vi "ProdaNG.ProcessStepResult.New.vi"(8 "error in (no error)":errorcluster, 10 "ProcessStepResult":T1, 11 "dbHandle":i32) -> (0 "error out":errorcluster, 2 "ProcessStepResult out":T1, 3 "dbHandle":i32)   [LabVIEW 2016]
doc: "This function creates a new record from a prefilled ProcessStepResult structure. Additionally the mdTime in the according product is set the current time and the mdProcessStepId is set to the created id.\nParameter:\nhandle is an Integer, which is returned by the function Login() at the creation of a new connection.\nprocessStepResult is a pointer on a ProcessStepResult structure, which elements must be prefilled. The structure must be defined and filled in the calling program. Nearly all elements of the structure must be set to reasonable values. The element id is filled by the DLL with a new Id for the created record, if the returncode is 0. The element startTime is filled automatically with the current time by the DLL and the endTime is deleted. \nThe element statusId is of particular importance:\nIf this element is passed with the value -1, the DLL automatically sets the standard status 2 (in Process), while otherwise the returned status is set.\n\nReturncodes:\n0 No error \n< 0 ORACLE Error code\n 6 (ERROR_INVALID_HANDLE) in case of an invalid handle"
uses:
  Controls/ProdaNG.ProcessStepResult.ctl
  Controls/ProdaNG.ProcessStepResultSize.ctl
  prodllNG.dll
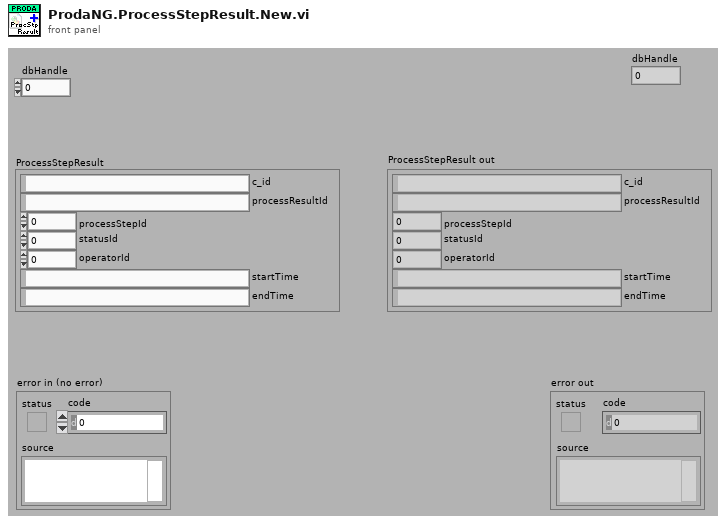
[diagram p1: front panel]
types:
  T1 = typedef "ProdaNG.ProcessStepResult.ctl" = cluster{"c_id":string, "processResultId":string, "processStepId":i32, "statusId":i32, "operatorId":i32, "startTime":string, "endTime":string}
  T2 = typedef "ProdaNG.ProcessStepResultSize.ctl" = cluster{"c_id":i32, "processResultId":i32, "processStepId":i32, "statusId":i32, "operatorId":i32, "startTime":i32, "endTime":i32}
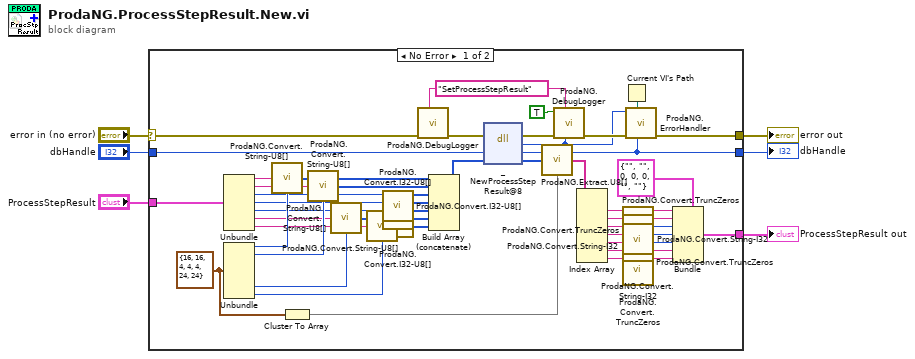
[diagram p0: block diagram]
diagram:
  n1 = case shown="No Error" "error in (no error)" {
    selector: "error in (no error)" -> [w31 w59]
    tunnel: [w28 w59] -> w5
    tunnel: "ProcessStepResult" -> [w29 _]
    tunnel: [w7 _] -> w3
    tunnel: "dbHandle" -> [w30 w58]
    tunnel: [w27 w58] -> w1
    frame No Error {
      w17 = T2 {"c_id"=16, "processResultId"=16, "processStepId"=4, "statusId"=4, "operatorId"=4, "startTime"=24, "endTime"=24} ("ProcessStepResultSize")
      w54 = "SetProcessStepResult" ("cmd")
      n2 = Unbundle(w29) -> ("c_id"=w56:string, "processResultId"=w57:string, "processStepId"=w44:i32, "statusId"=w43:i32, "operatorId"=w34:i32, "startTime"=w39:string, "endTime"=w38:string)
      n3 = Unbundle(w17) -> ("c_id"=w48:i32, "processResultId"=w46:i32, "startTime"=w33:i32, "endTime"=w32:i32)  [unwired: 3 out]
      n4 = call "ProdaNG.Convert.String-U8[].vi"("Input String"=w56, "Size"=w48) -> ("Output"=w47:u8[])
      n5 = Cluster To Array(cluster=w17) -> (array=w18:i32[])
      n6 = call "ProdaNG.Convert.String-U8[].vi"("Input String"=w57, "Size"=w46) -> ("Output"=w45:u8[])
      n7 = call "ProdaNG.Convert.String-U8[].vi"("Input String"=w39, "Size"=w33) -> ("Output"=w36:u8[])
      n8 = call "ProdaNG.Convert.String-U8[].vi"("Input String"=w38, "Size"=w32) -> ("Output"=w37:u8[])
      n9 = call "ProdaNG.Convert.I32-U8[].vi"("32bit integer"=w44) -> ("unsigned byte array"=w42:u8[])  [unwired: 10 in]
      n10 = call "ProdaNG.Convert.I32-U8[].vi"("32bit integer"=w43) -> ("unsigned byte array"=w41:u8[])  [unwired: 10 in]
      n11 = call "ProdaNG.Convert.I32-U8[].vi"("32bit integer"=w34) -> ("unsigned byte array"=w35:u8[])  [unwired: 10 in]
      n12 = call "ProdaNG.DebugLogger.vi"("cmd"=w54, "error in (no error)"=w31) -> ("error out"=w49:errorcluster)  [unwired: 9 in]
      n13 = Build Array (concatenate)(w47, w45, w42, w41, w35, w36, w37) -> (w40:u8[])
      n14 = dll-call lib="D:/svn/LineTraceSystem/SOFTWARE/sources/Database/ProdaNG/prodllNG.dll" fn="_NewProcessStepResult@8" ("ProDll.dll:InitProDll")(error in=w49, "dbHandle"=w30, "processResult"=w40) -> (error out=w52:errorcluster, "return type"=w50:i32, "dbHandle"=w27:i32, "processResult"=w19:u8[])  [unwired: 2 in, 1 out]
      n15 = call "ProdaNG.Extract.U8[].vi"("unsigned byte array"=w19, "Sizes"=w18) -> ("Elements"=w16:string[])
      n16 = call "ProdaNG.DebugLogger.vi"("return type"=w50, "cmd"=w54, "error in (no error)"=w52, "done? (F)"=TRUE) -> ("error out"=w51:errorcluster)  [unwired: 7 in]
      n17 = Index Array(array=w16) -> (element #1=w21:string, element #2=w20:string, element #3=w26:string, element #4=w10:string, element #5=w9:string, element #6=w11:string, element #7=w14:string)  [unwired: 7 in]
      n18 = Current VI's Path() -> (path=w55:path)
      n19 = call "ProdaNG.Convert.TruncZeros.vi"("string with \\0s"=w21) -> ("LV string"=w23:string)  [unwired: 10 in]
      n20 = call "ProdaNG.Convert.TruncZeros.vi"("string with \\0s"=w20) -> ("LV string"=w22:string)  [unwired: 10 in]
      n21 = call "ProdaNG.Convert.String-I32.vi"("unsigned byte string"=w26) -> ("32bit integer"=w25:i32)  [unwired: 10 in]
      n22 = call "ProdaNG.Convert.String-I32.vi"("unsigned byte string"=w10) -> ("32bit integer"=w24:i32)  [unwired: 10 in]
      n23 = call "ProdaNG.Convert.String-I32.vi"("unsigned byte string"=w9) -> ("32bit integer"=w8:i32)  [unwired: 10 in]
      n24 = call "ProdaNG.Convert.TruncZeros.vi"("string with \\0s"=w11) -> ("LV string"=w12:string)  [unwired: 10 in]
      n25 = call "ProdaNG.Convert.TruncZeros.vi"("string with \\0s"=w14) -> ("LV string"=w13:string)  [unwired: 10 in]
      n26 = call "ProdaNG.ErrorHandler.vi"("dbHandleIn"=w27, "Path"=w55, "error in"=w51, "output_parameter"=w50) -> ("error out"=w28:errorcluster)  [unwired: 7 in]
      n27 = Bundle(cluster=T1 {"c_id"="", "processResultId"="", "processStepId"=0, "statusId"=0, "operatorId"=0, "startTime"="", "endTime"=""} ("ProcessStepResult out"), "c_id"=w23, "processResultId"=w22, "processStepId"=w25, "statusId"=w24, "operatorId"=w8, "startTime"=w12, "endTime"=w13) -> (w7:T1)
    }
    frame Error {
    }
  }
  "error out" <- w5
  "ProcessStepResult out" <- w3
  "dbHandle" <- w1
